vi "Write TCPIP connection ID.vi"(8 "error in (no error)":errorcluster, 10 "TCPIP connection ID":refnum<k5>, 11 "Client Proxy LNA in":refnum<class "Client Proxy LNA.lvclass">) -> (0 "error out":errorcluster, 3 "Client Proxy LNA out":refnum<class "Client Proxy LNA.lvclass">)   [LabVIEW 2016, in "Client Proxy LNA.lvlib" / "Client Proxy LNA.lvclass"]
uses:
  Client Proxy LNA.lvclass
  Client Proxy LNA.lvclass/Client Proxy LNA.ctl
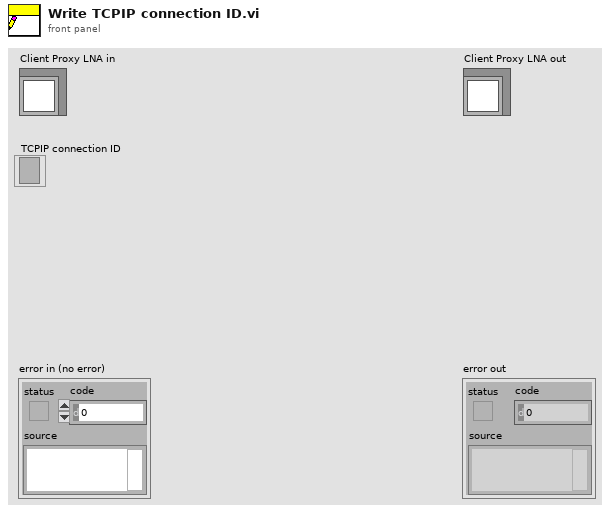
[diagram p1: front panel]
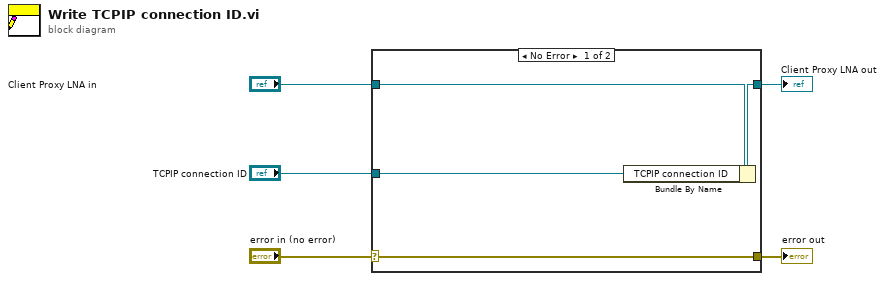
[diagram p0: block diagram]
diagram:
  n1 = case shown="No Error" "error in (no error)" {
    selector: "error in (no error)" -> [w9 w10]
    tunnel: [w9 w10] -> w4
    tunnel: [w7 w11] -> w2
    tunnel: "Client Proxy LNA in" -> [w8 w11]
    tunnel: "TCPIP connection ID" -> [w6 _]
    frame No Error {
      n2 = Bundle By Name(cluster=w8, "TCPIP connection ID"=w6) -> (w7:refnum<class "Client Proxy LNA.lvclass">)
    }
    frame Error {
    }
  }
  "error out" <- w4
  "Client Proxy LNA out" <- w2
